vi "Refresh Stats.vi"(8 "error in (no error)":errorcluster, 11 "CIFCorePlugin in":refnum<class "CIFCorePlugin.lvclass">) -> (0 "error out":errorcluster, 3 "CIFCorePlugin out":refnum<class "CIFCorePlugin.lvclass">)   [LabVIEW 2021, in "CIFCorePlugin.lvclass"]
uses:
  CIFCorePlugin.lvclass
  CIFCorePlugin.lvclass/CIFCorePlugin.ctl
  CIFCoreCommon/Typedef/Timing Stats Base.ctl
  CIFCoreCommon/CIFCoreCommon.lvlib
  CIFCoreCommon/Typedef/Timing Statistics.ctl
  CIFCoreCommon/Typedef/Simple Error.ctl
  CIFCoreCommon/Typedef/FIFO Statistics.ctl
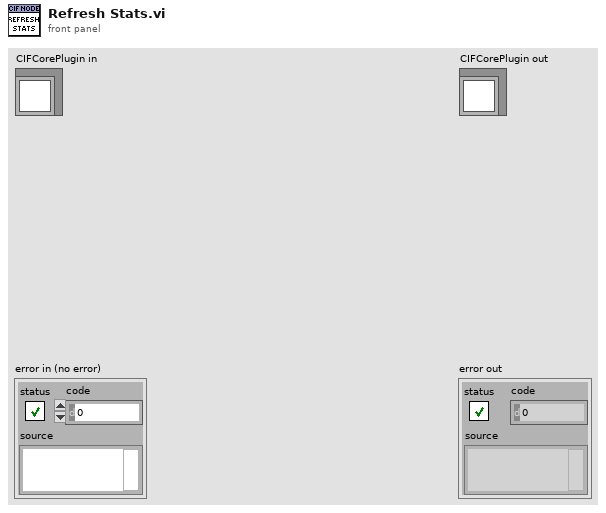
[diagram p1: front panel]
types:
  T1 = typedef "CIFCoreCommon.lvlib/FIFO Statistics.ctl" = cluster{"From T0":T2, "From Previous Plugin":T2, "Output Error":T2}
  T2 = typedef "CIFCoreCommon.lvlib/Timing Stats Base.ctl" = cluster{"Max":i32, "Min":i32}
  T3 = typedef "CIFCoreCommon.lvlib/Simple Error.ctl" = cluster{"status":bool, "code":i32}
  T4 = typedef "CIFCoreCommon.lvlib/Timing Statistics.ctl" = cluster{"Period":T2, "Wake Error":T2, "Execute":T2, "Housekeep":T2, "Idle":T2}
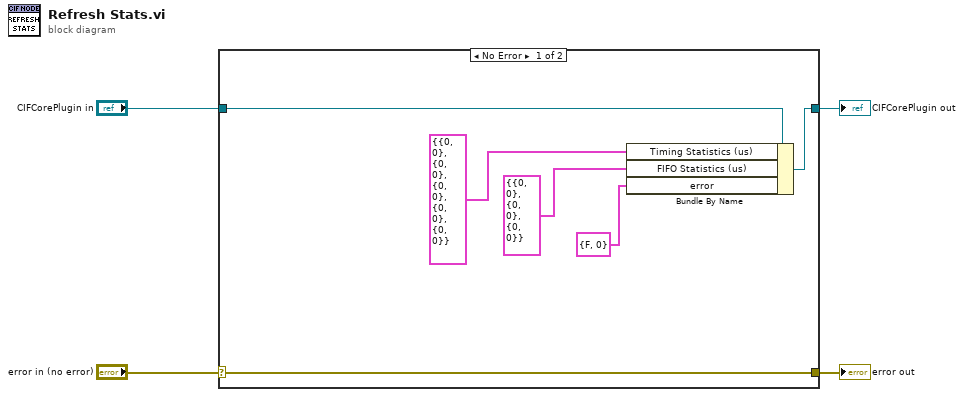
[diagram p0: block diagram]
diagram:
  n1 = case shown="No Error" "error in (no error)" {
    selector: "error in (no error)" -> [w10 w12]
    tunnel: [w10 w12] -> w3
    tunnel: [w8 w11] -> w1
    tunnel: "CIFCorePlugin in" -> [w9 w11]
    frame No Error {
      n2 = Bundle By Name(cluster=w9, "Timing Statistics (us)"=T4 {"Period"={"Max"=0, "Min"=0}, "Wake Error"={"Max"=0, "Min"=0}, "Execute"={"Max"=0, "Min"=0}, "Housekeep"={"Max"=0, "Min"=0}, "Idle"={"Max"=0, "Min"=0}} ("Status.Timing Statistics (us)"), "FIFO Statistics (us)"=T1 {"From T0"={"Max"=0, "Min"=0}, "From Previous Plugin"={"Max"=0, "Min"=0}, "Output Error"={"Max"=0, "Min"=0}} ("Status.FIFO Statistics (us)"), "error"=T3 {"status"=FALSE, "code"=0} ("Status.error")) -> (w8:refnum<class "CIFCorePlugin.lvclass">)
    }
    frame Error {
    }
  }
  "error out" <- w3
  "CIFCorePlugin out" <- w1
